vi "Read Show Window.vi"(8 "error in (no error)":errorcluster, 11 "MDI serialize in":refnum<class "MDI serialize.lvclass">) -> (0 "error out":errorcluster, 2 "Show?":bool, 3 "MDI serialize out":refnum<class "MDI serialize.lvclass">)   [LabVIEW 2019, in "MDI serialize.lvclass"]
uses:
  MDI serialize.lvclass
  MDI serialize.lvclass/MDI serialize.ctl
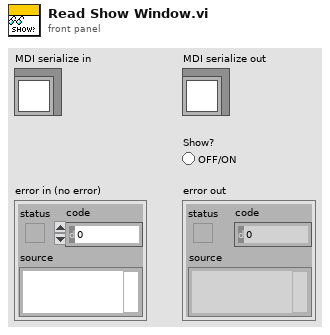
[diagram p1: front panel]
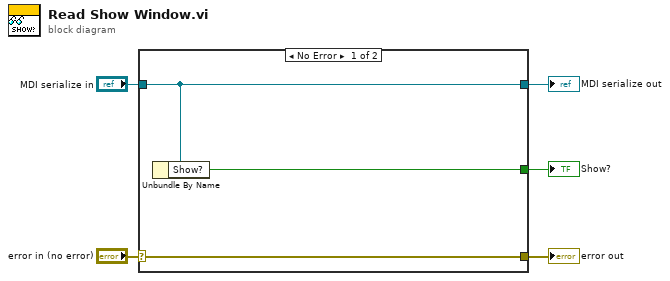
[diagram p0: block diagram]
diagram:
  n1 = case shown="No Error" "error in (no error)" {
    selector: "error in (no error)" -> [w8 w9]
    tunnel: [w8 w9] -> w4
    tunnel: [w7 w10] -> w2
    tunnel: "MDI serialize in" -> [w7 w10]
    tunnel: [w6 _] -> w1
    frame No Error {
      n2 = Unbundle By Name(w7) -> ("Show?"=w6:bool)
    }
    frame Error {
    }
  }
  "error out" <- w4
  "MDI serialize out" <- w2
  "Show?" <- w1
